vi "adam-read-&-parse-thermocouples.vi"(7 "Thermocouples in":T1, 8 "error in (no error)":errorcluster, 9 "Bytes at Port":u32, 11 "VISA Refnum in":refnum<visa-resource-name>) -> (0 "error out":errorcluster, 1 "status  out":string, 2 "read buffer":string, 3 "VISA Refnum out":refnum<visa-resource-name>, 4 "acknowledge char":string, 5 "Thermocouples out":T1)   [LabVIEW 2024]
uses:
  controls/depreciated/thermocouple-data-cluster.ctl
panel:
  out "read return":u32
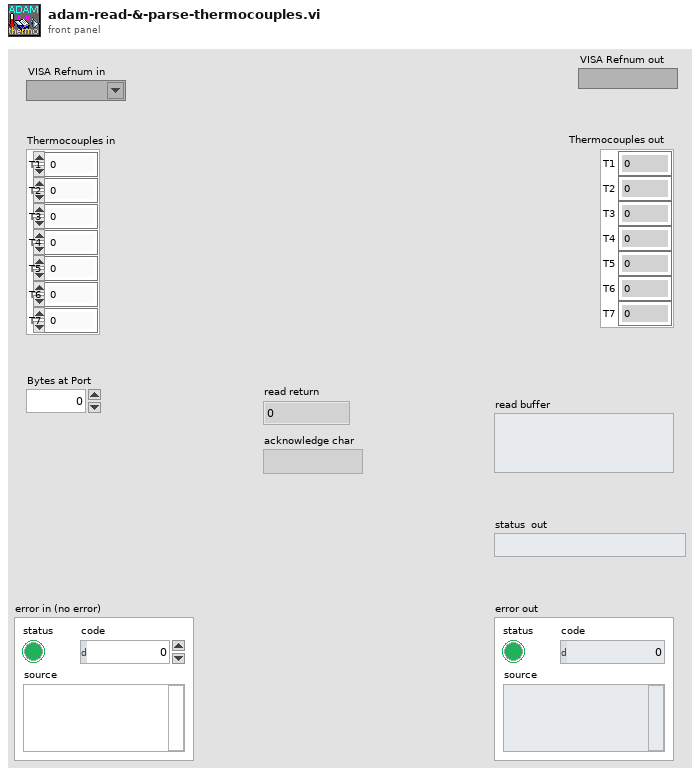
[diagram p1: front panel]
types:
  T1 = typedef "thermocouple-data-cluster.ctl" = cluster{"T1":dbl, "T2":dbl, "T3":dbl, "T4":dbl, "T5":dbl, "T6":dbl, "T7":dbl}
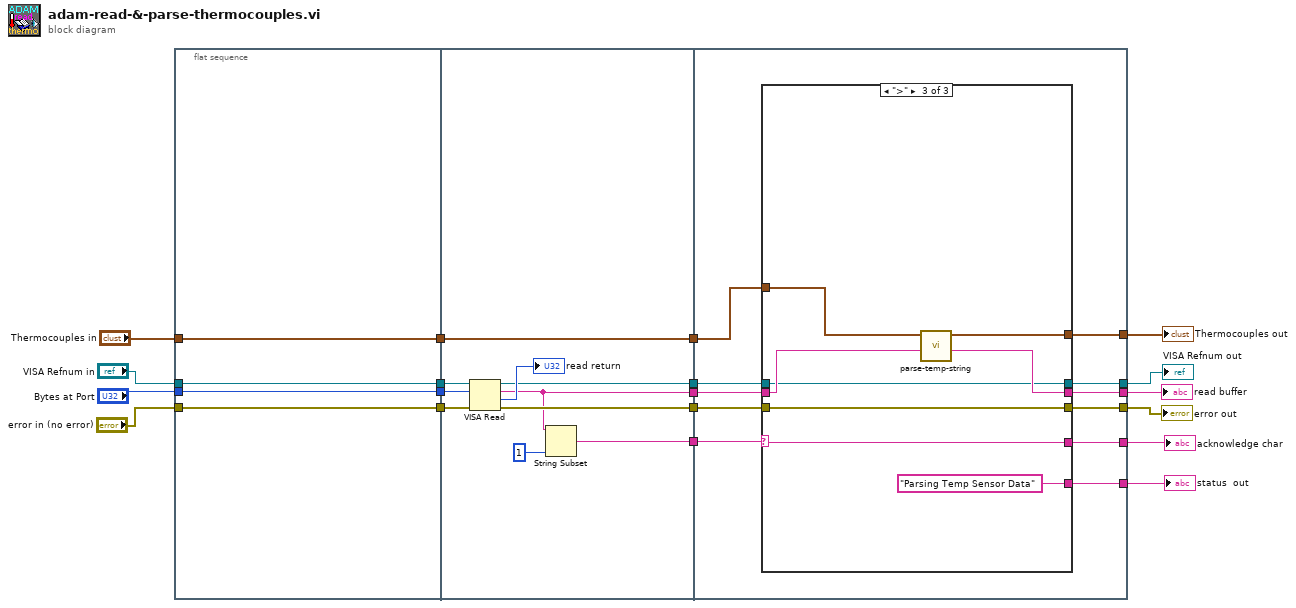
[diagram p0: block diagram]
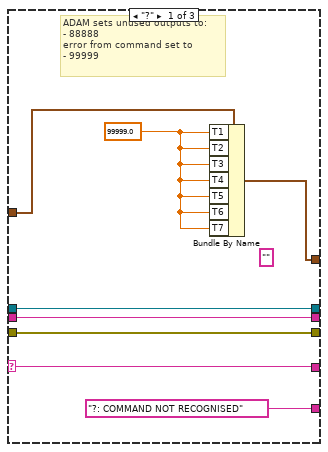
[diagram p2: hidden frame]
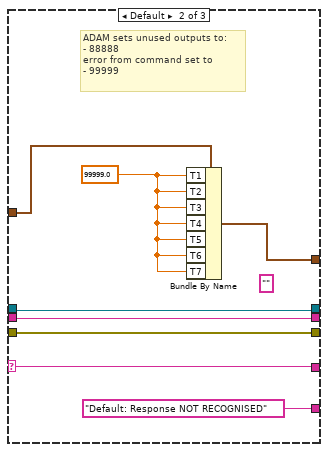
[diagram p3: hidden frame]
diagram:
  n1 = flat-sequence {
    tunnel: [w23] -> w19
    tunnel: "VISA Refnum in" -> [w23]
    tunnel: [w22] -> w17
    tunnel: "Bytes at Port" -> [w22]
    tunnel: [w21] -> w15
    tunnel: "error in (no error)" -> [w21]
    tunnel: [w20] -> w13
    tunnel: "Thermocouples in" -> [w20]
    tunnel: w19 -> [w27]
    tunnel: w17 -> [w26]
    tunnel: w15 -> [w25]
    tunnel: w13 -> [w24]
    tunnel: [w31] -> w11
    tunnel: [w30] -> w10
    tunnel: [w29] -> w9
    tunnel: [w28] -> w8
    tunnel: [w24] -> w7
    tunnel: w11 -> [w35]
    tunnel: w10 -> [w36]
    tunnel: w9 -> [w43]
    tunnel: w8 -> [w44]
    tunnel: w7 -> [w42]
    tunnel: [w41] -> w6
    tunnel: [w40] -> w5
    tunnel: [w39] -> w4
    tunnel: [w38] -> w3
    tunnel: [w37] -> w2
    tunnel: [w34] -> w1
    frame #0 {
    }
    frame #1 {
      n2 = VISA Read(VISA resource name=w27, byte count=w26, error in (no error)=w25) -> (VISA resource name out=w28:refnum<visa-resource-name>, read buffer=w29:string, return count=→"read return":u32, error out=w30:errorcluster)
      n3 = String Subset(string=w29, length (rest)=1 ("length (rest)")) -> (substring=w31:string)  [unwired: 1 in]
    }
    frame #2 {
      n4 = case shown="\">\"" w35 {
        selector: w35 -> [w45 w53 w61]
        tunnel: [w51 w59 w67] -> w41
        tunnel: [w52 w60 w64] -> w40
        tunnel: [w50 w58 w63] -> w39
        tunnel: [w47 w54 w66] -> w38
        tunnel: ["?: COMMAND NOT RECOGNISED" ("status") "Default: Response NOT RECOGNISED" ("status") "Parsing Temp Sensor Data" ("status")] -> w37
        tunnel: w44 -> [w52 w60 w64]
        tunnel: w36 -> [w50 w58 w63]
        tunnel: w43 -> [w51 w59 w68]
        tunnel: w42 -> [w46 w55 w62]
        tunnel: [w45 w53 w61] -> w34
        frame "?" {
          w48 = 99999.0 ("T1")
          (unwired) "" ("csv")
          # "ADAM sets unused outputs to:\n- 88888\nerror from command set to\n- 99999"
          n5 = Bundle By Name(cluster=w46, "T1"=w48, "T2"=w48, "T3"=w48, "T4"=w48, "T5"=w48, "T6"=w48, "T7"=w48) -> (w47:T1)
        }
        frame Default {
          w56 = 99999.0 ("T1")
          (unwired) "" ("csv")
          # "ADAM sets unused outputs to:\n- 88888\nerror from command set to\n- 99999"
          n6 = Bundle By Name(cluster=w55, "T1"=w56, "T2"=w56, "T3"=w56, "T4"=w56, "T5"=w56, "T6"=w56, "T7"=w56) -> (w54:T1)
        }
        frame ">" {
          n7 = call "parse-temp-string.vi"("read buffer in"=w68, "Thermocouples"=w62) -> ("csv"=w67:string, "Thermocouples"=w66:T1)  [unwired: 8 in]
        }
      }
    }
  }
  "status  out" <- w2
  "Thermocouples out" <- w3
  "VISA Refnum out" <- w5
  "read buffer" <- w6
  "error out" <- w4
  "acknowledge char" <- w1
